vi "Skeleton_Virtual_Instrument.vi"() -> ()   [LabVIEW 2014]
uses:
  <vilib>/addons/control/pid/NI_PID_autopid.lvlib
panel:
  in  "autotune? (F)":bool
  out "Temperature":dbl(graph)
  in  "Volume":dbl
  out "steps (seg)":dbl
  in  "Step motor stop max 2000":dbl=1900.0
  in  "Output range":cluster{"Output high":dbl, "Output low":dbl}={"Output high"=100.0, "Output low"=0.0} {"Output low" format="%.2f"; "Output high" format="%.2f"}
  out "Output":dbl(graph)
  out "Low Limit":bool
  out "High Limit":bool
  in  "Alarm":cluster{dbl, dbl}(slide)={0.8235294117647058, 12.444444444444443} scale=0.0..14.0
  out "MV:":dbl(slide)=100.0 scale=-100.0..100.0
  in  "SP:":dbl(slide)=1.205298013245033 min=0.0 max=0.0 scale=0.0..14.0
  out "PV:":dbl(slide)=33.01408837398299 scale=0.0..14.0
  in  "PID gains":T1={"proportional gain (Kc)"=25.0, "integral time (Ti, min)"=0.008, "derivative time (Td, min)"=0.001} {"derivative time (Td, min)" format="%.3f"; "integral time (Ti, min)" format="%.3f"; "proportional gain (Kc)" format="%.3f"}
  out "Monitoring System of Chemical Modification of Starches":cluster{"initial PV":dbl, "SP:":dbl, dbl, dbl}(graph)
  in  "Fast sampling  = 1, slow > 1":i32=1 min=1 max=1000 step=1
  out "Numeric":dbl
  in  "error IO":errorcluster
  in  "flow control":u16(ring) items=["None"=0, "XON/XOFF"=1, "RTS/CTS"=2, "DTR/DSR"=4]
  in  "stop bits":u16(ring)=10 items=["1.0"=10, "1.5"=15, "2.0"=20]
  in  "parity":u16(ring) items=["None", "Odd", "Even", "Mark", "Space"]
  in  "data bits":u16=8 min=5 max=8 step=1
  in  "bytes to read":u32=26
  in  "VISA resource name":refnum<visa-resource-name>="COM1"
  in  "baud rate":u32=9600
  out "pH":dynamicdata(graph)
  out "?":dbl
  out "?":dbl
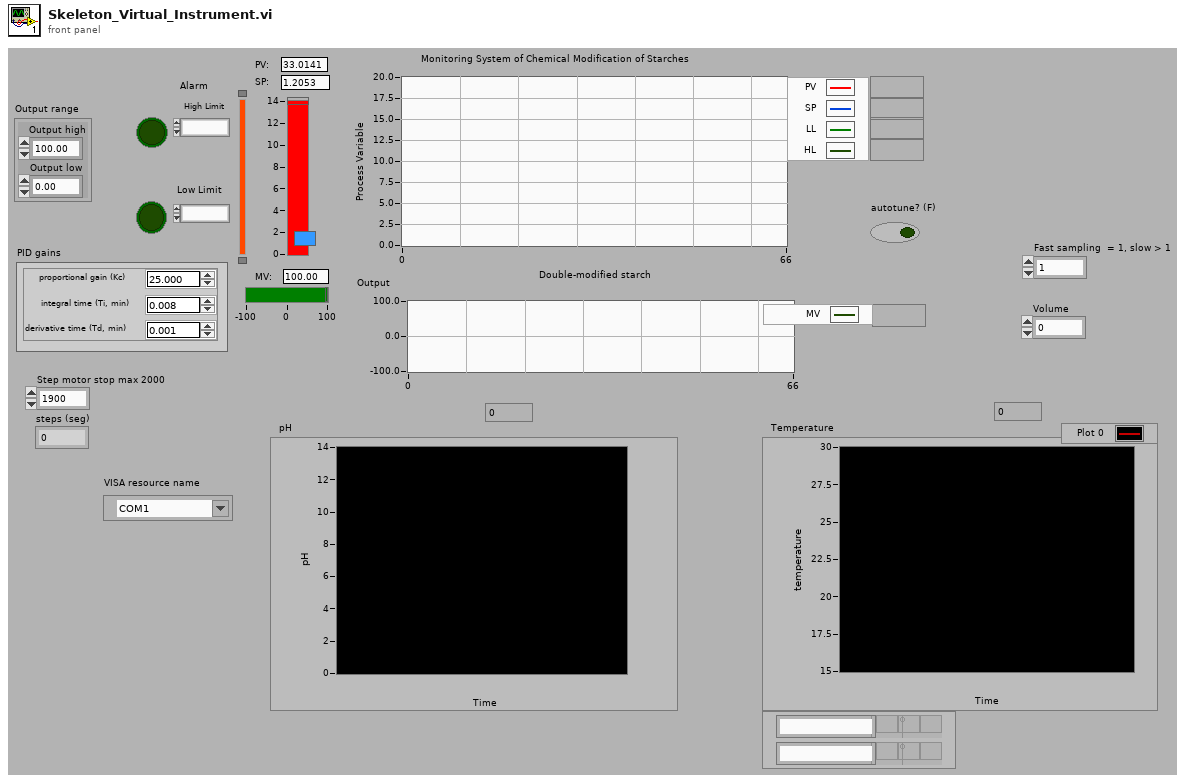
[diagram p1: front panel]
types:
  T1 = cluster{"proportional gain (Kc)":dbl, "integral time (Ti, min)":dbl, "derivative time (Td, min)":dbl}
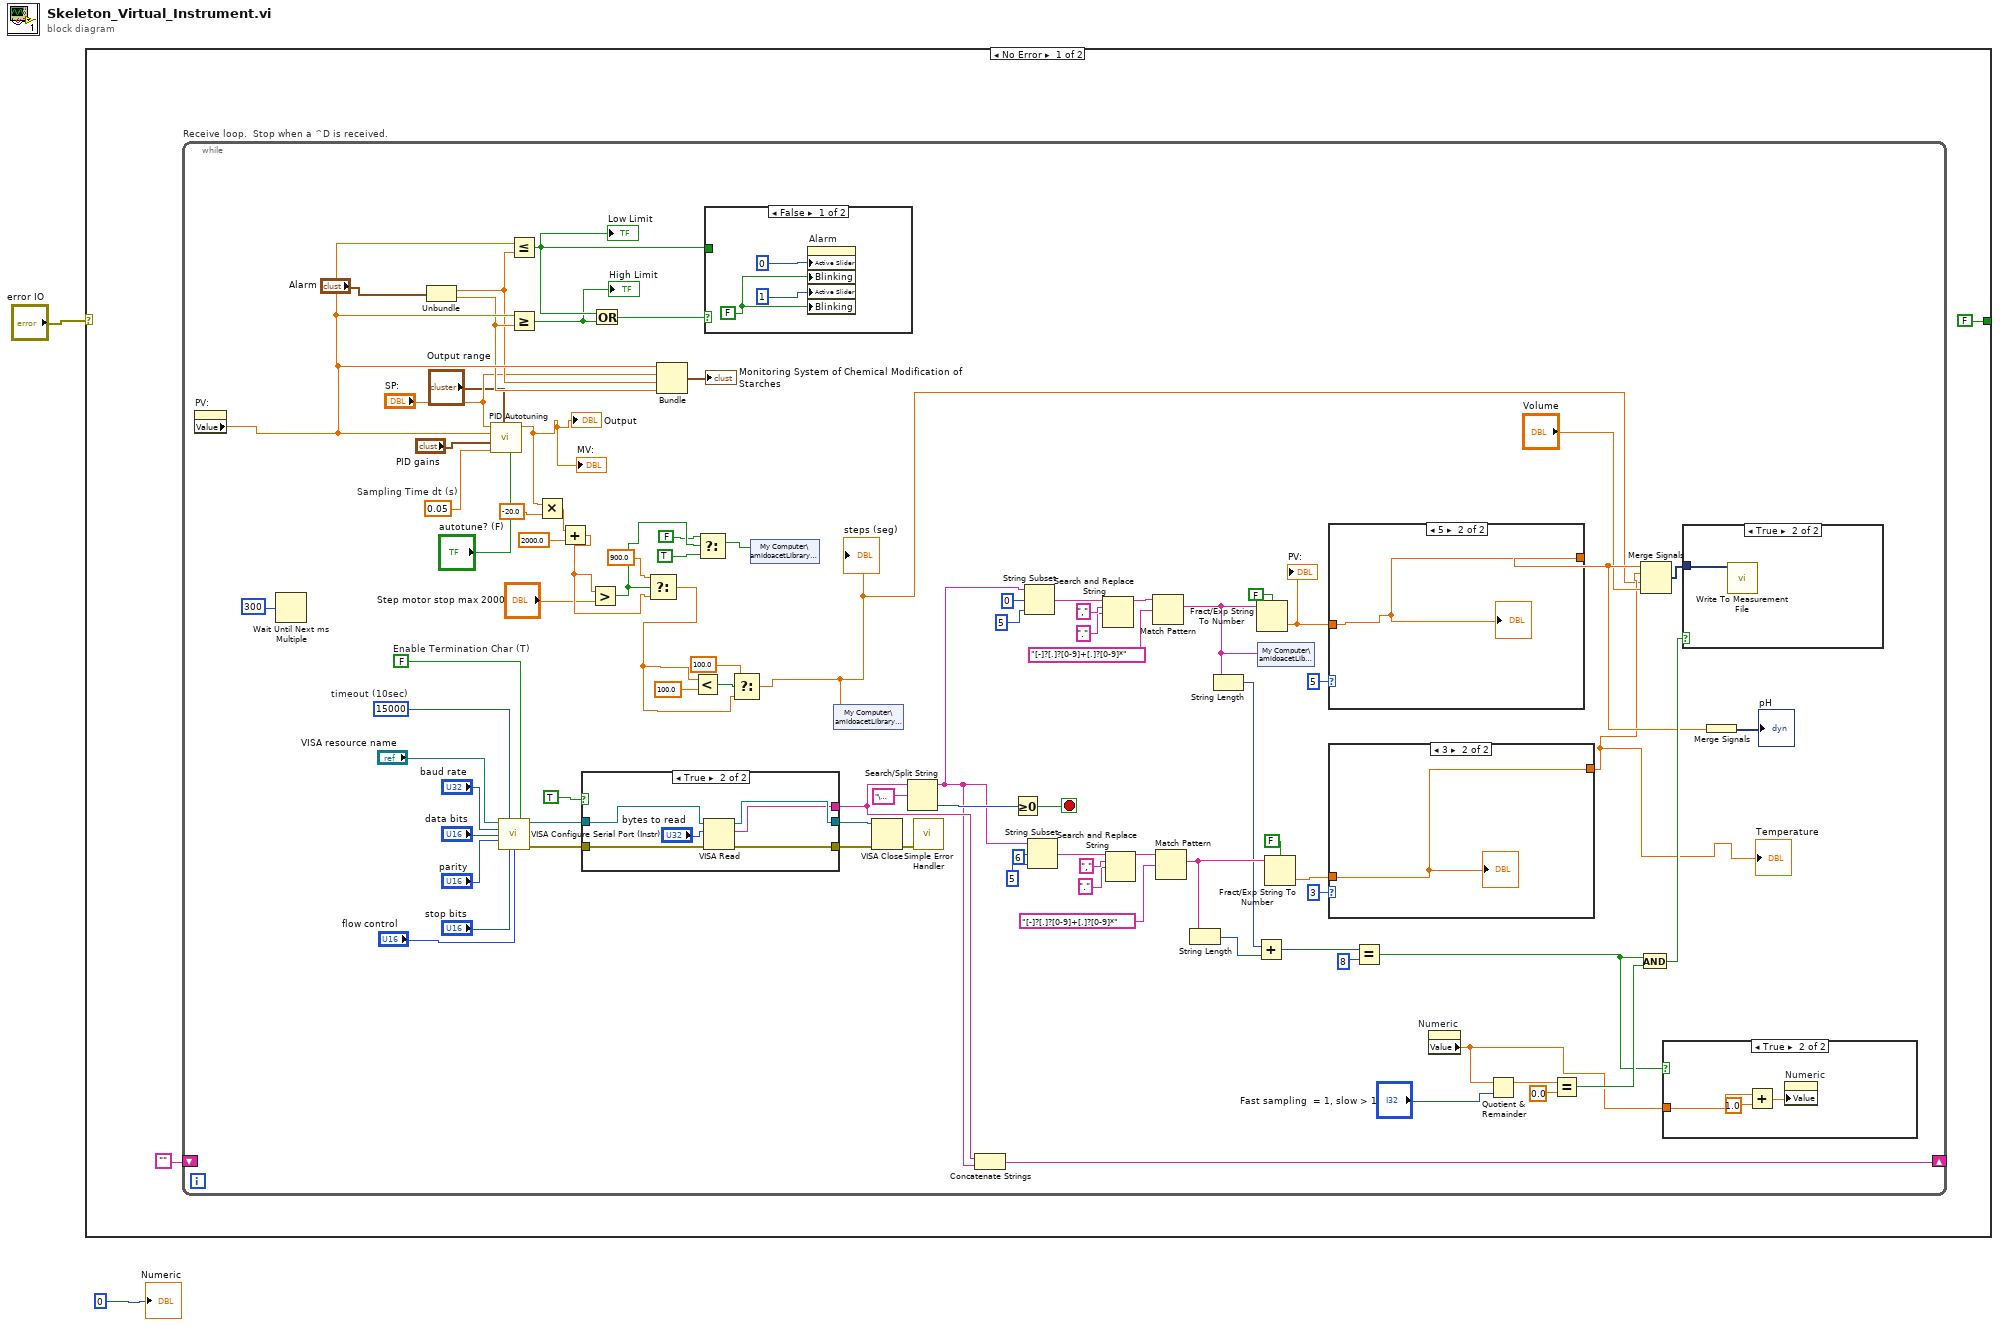
[diagram p0: block diagram]
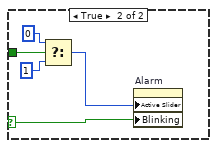
[diagram p2: hidden frame]
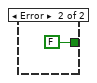
[diagram p8: hidden frame]
diagram:
  n1 = case shown="No Error" "error IO" {
    tunnel: [FALSE FALSE] -> _
    frame No Error {
      n2 = while "Receive loop.  Stop when a ^D is received." {
        shift-left: "" -> [_]
        shift-right: [w60] -> _
        stop <- w61 stop-if-true
        w37 = 0.05  # Sampling Time dt (s)
        w72 = FALSE  # Enable Termination Char (T)
        w71 = u32 15000  # timeout (10sec)
        n3 = property on="PV:" class="Slide (strict)"() -> ("Value"=w38:dbl)  [unwired: 2 in, 2 out]
        n4 = Wait Until Next ms Multiple(millisecond multiple=u32 300) -> ()  [unwired: 1 out]
        n5 = Unbundle("Alarm") -> (w32:dbl, w33:dbl)
        n6 = call <vilib>:"PID Autotuning.vi"("autotune? (F)"="autotune? (F)", "output range"="Output range", "dt (s)"=w37, "PID gains"="PID gains", "process variable"=w38, "setpoint"="SP:") -> ("output"=w12:dbl)  [unwired: 2 in, 3 out]
        "MV:" <- w12
        "Output" <- w12
        n7 = call-poly <vilib>:"VISA Configure Serial Port (Instr).vi"("VISA resource name"="VISA resource name", "timeout (10sec)"=w71, "Enable Termination\nChar (T)"=w72, "baud rate (9600)"="baud rate", "data bits (8)"="data bits", "parity (0:none)"="parity", "stop bits (10: 1 bit)"="stop bits", "flow control (0:none)"="flow control") -> ("VISA resource name out"=w76:refnum<visa-resource-name>, "error out"=w77:errorcluster)  [unwired: 6 in]
        n8 = Less Or Equal?(x=w38, y=w32) -> (x <= y?=w36:bool)
        "Low Limit" <- w36
        n9 = Greater Or Equal?(x=w38, y=w33) -> (x >= y?=w34:bool)
        "High Limit" <- w34
        n10 = Multiply(x=w12, y=-20.0 ("x")) -> (x*y=w22:dbl)
        n11 = Add(x=w22, y=2000.0) -> (x+y=w19:dbl)
        n12 = case shown="True" TRUE ("Aquisicao  dos dados") {
          tunnel: w77 -> [w105 w108]
          tunnel: [w105 w111] -> w67
          tunnel: [w104 w110] -> w68
          tunnel: w76 -> [w104 w107]
          tunnel: [_ w106] -> w59
          frame False {
          }
          frame True {
            n13 = VISA Read(VISA resource name=w107, byte count="bytes to read", error in (no error)=w108) -> (VISA resource name out=w110:refnum<visa-resource-name>, read buffer=w106:string, error out=w111:errorcluster)  [unwired: 1 out]
          }
        }
        n14 = Greater?(x=w19, y="Step motor stop max 2000") -> (0:w8:bool)
        n15 = Or(x=w36, y=w34) -> (x .or. y?=w35:bool)
        n16 = Select(t=900.0 ("y"), s=w8, f=w19) -> (s? t:f=w14:dbl)
        n17 = Bundle("Value"=w38, "SP:"="SP:", w32, w33) -> (→"Monitoring System of Chemical Modification of Starches":cluster{"Value":dbl, "SP:":dbl, dbl, dbl})  [unwired: 1 in]
        n18 = Less?(x=w14, y=100.0) -> (x < y?=w17:bool)
        n19 = Select(t=FALSE, s=w8, f=TRUE) -> (s? t:f=w9:bool)
        n20 = case shown="False" w35 {
          selector: w35 -> [_ w100]
          tunnel: w36 -> [_ w96]
          frame False {
            w94 = FALSE ("Blinking")
            n21 = property on="Alarm" class="Slide (strict)"("Active Slider"=0, "Blinking"=w94, "Active Slider"=1, "Blinking"=w94) -> ()  [unwired: 2 in, 2 out]
          }
          frame True {
            n22 = Select(t=0 ("Active Slider"), s=w96, f=1 ("Active Slider")) -> (s? t:f=w99:i32)
            n23 = property on="Alarm" class="Slide (strict)"("Active Slider"=w99, "Blinking"=w100) -> ()  [unwired: 2 in, 2 out]
          }
        }
        n24 = Select(t=100.0, s=w17, f=w14) -> (s? t:f=w10:dbl)
        "steps (seg)" <- w10
        n25 = shared-variable "My Computer\\amidoacetLibrary.lvlib\\STOP"(w9) -> ()  [unwired: 1 in, 1 out]
        n26 = shared-variable "My Computer\\amidoacetLibrary.lvlib\\steps"(w10) -> ()  [unwired: 1 in, 1 out]
        n27 = VISA Close(VISA resource name=w68, error in (no error)=w67) -> (error out=w69:errorcluster)
        n28 = Search/Split String(string=w59, search string/char (-)="\u0004") -> (substring before match=w42:string, offset of match=w62:i32)  [unwired: 1 in, 1 out]
        n29 = call <vilib>:"Simple Error Handler.vi"("error in (no error)"=w69) -> ()  [unwired: 4 in, 5 out]
        n30 = Concatenate Strings(w59, w42) -> (w60:string)
        n31 = Greater Or Equal To 0?(x=w62) -> (x >= 0?=w61:bool)
        n32 = String Subset(string=w42, offset (0)=0, length (rest)=5 ("offset (0)")) -> (substring=w52:string)
        n33 = String Subset(string=w42, offset (0)=6, length (rest)=5 ("offset (0)")) -> (substring=w46:string)
        n34 = Search and Replace String(input string=w52, search string=",", replace string=".") -> (result string=w49:string)  [unwired: 5 in, 3 out]
        n35 = Search and Replace String(input string=w46, search string=",", replace string=".") -> (result string=w45:string)  [unwired: 5 in, 3 out]
        n36 = Match Pattern(string=w49, regular expression="[-]?[.]?[0-9]+[.]?[0-9]*") -> (match substring=w39:string)  [unwired: 1 in, 3 out]
        n37 = Match Pattern(string=w45, regular expression="[-]?[.]?[0-9]+[.]?[0-9]*") -> (match substring=w83:string)  [unwired: 1 in, 3 out]
        n38 = String Length(string=w83) -> (length=w80:i32)
        n39 = String Length(string=w39) -> (length=w81:i32)
        n40 = Add(x=w81, y=w80) -> (x+y=w79:i32)
        n41 = Fract/Exp String To Number(use system decimal point (T)=FALSE, string=w39) -> (number=w26:dbl)  [unwired: 2 in, 1 out]
        "PV:" <- w26
        n42 = shared-variable "My Computer\\amidoacetLibrary.lvlib\\pH"(w39) -> ()  [unwired: 1 in, 1 out]
        n43 = Fract/Exp String To Number(use system decimal point (T)=FALSE, string=w83) -> (number=w82:dbl)  [unwired: 2 in, 1 out]
        n44 = case shown="5" 5 {
          tunnel: w26 -> [_ w113]
          tunnel: [_ w113] -> w40
          frame 0, Default {
          }
          frame 5 {
            "?" <- w113
          }
        }
        n45 = case shown="3" 3 {
          tunnel: w82 -> [_ w114]
          tunnel: [_ w114] -> w11
          frame 0, Default {
          }
          frame 3 {
            "?" <- w114
          }
        }
        "Temperature" <- w11
        n46 = Equal?(x=w79, y=8) -> (x = y?=w53:bool)
        n47 = property on="Numeric" class="DigNum (strict)"() -> ("Value"=w54:dbl)  [unwired: 2 in, 2 out]
        n48 = Quotient & Remainder(x=w54, y="Fast sampling  = 1, slow > 1") -> (x-y*floor(x/y)=w58:dbl)  [unwired: 1 out]
        n49 = Equal?(x=w58, y=0.0) -> (x = y?=w56:bool)
        n50 = And(x=w53, y=w56) -> (x .and. y?=w55:bool)
        n51 = Merge Signals(w40, w11, w10, "Volume") -> (w44:dynamicdata)
        n52 = case shown="True" w53 {
          tunnel: w54 -> [_ w101]
          frame False {
          }
          frame True {
            n53 = Add(x=w101, y=1.0) -> (x+y=w102:dbl)
            n54 = property on="Numeric" class="DigNum (strict)"("Value"=w102) -> ()  [unwired: 2 in, 2 out]
          }
        }
        n55 = case shown="True" w55 {
          tunnel: w44 -> [_ w112]
          frame False {
          }
          frame True {
            n56 = call "Write To Measurement File"("Signals"=w112) -> ()  [unwired: 16 in, 3 out]
          }
        }
        n57 = Merge Signals(w40) -> (→"pH":dynamicdata)
      }
    }
    frame Error {
    }
  }
  "Numeric" <- 0
